vi "Convert X & Y to polar degrees 0 to 360.vi"(8 "error in (no error)":errorcluster, 9 "y":dbl format="%0.2f", 11 "x":dbl format="%0.2f") -> (0 "error out":errorcluster, 2 "degree CCW x axis":dbl, 3 "R":dbl format="%0.2f")   [LabVIEW 2011]
doc: "Does conversion of x and y to polar, with angle in deg and wiht ranbge 0 to 360 CCW from x axis."
uses:
  <vilib>/ptbypt/NI_PtbyPt.lvlib
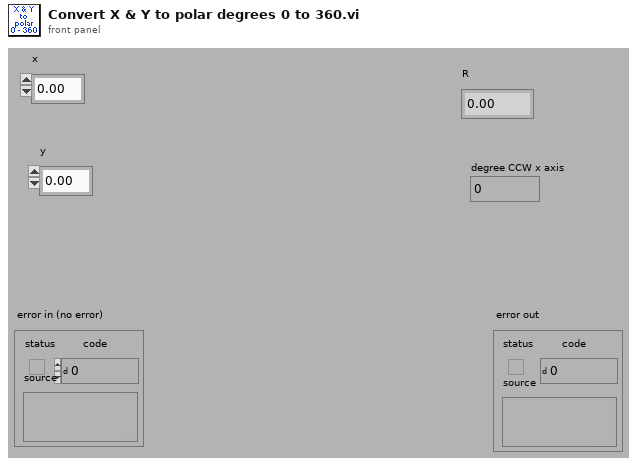
[diagram p1: front panel]
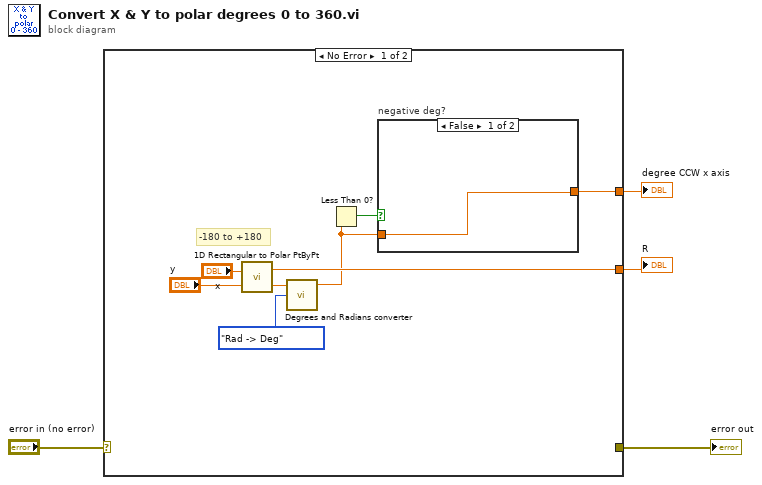
[diagram p0: block diagram]
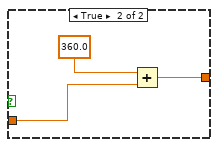
[diagram p2: hidden frame]
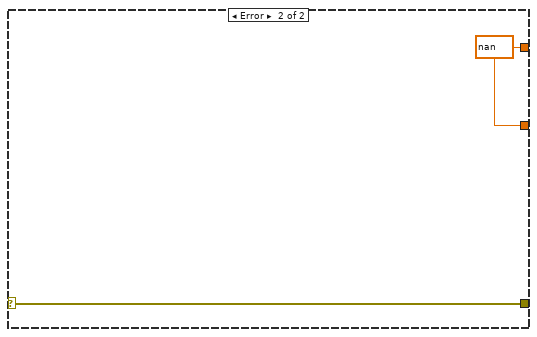
[diagram p3: hidden frame]
diagram:
  n1 = case shown="No Error" "error in (no error)" {
    selector: "error in (no error)" -> [_ w18]
    tunnel: [_ w18] -> w3
    tunnel: [w8 w17] -> w2
    tunnel: [w5 w17] -> w1
    frame No Error {
      # "-180 to +180"
      n2 = call <vilib>:"1D Rectangular to Polar PtByPt.vi"("y"="y", "x"="x") -> ("phase"=w12:dbl, "magnitude"=w8:dbl)
      n3 = call "Degrees and Radians converter.vi"("Units"=enum16{"Deg -> Rad", "Rad -> Deg"}."Rad -> Deg", "Angle IN"=w12) -> ("Angle Out"=w6:dbl)  [unwired: 3 in]
      n4 = Less Than 0?(x=w6) -> (x < 0?=w7:bool)
      n5 = case "negative deg?" shown="False" w7 {
        tunnel: w6 -> [w13 w16]
        tunnel: [w13 w14] -> w5
        frame False {
        }
        frame True {
          n6 = Add(x=360.0 ("y"), y=w16) -> (x+y=w14:dbl)
        }
      }
    }
    frame Error {
      w17 = nan ("Angle Out")
    }
  }
  "error out" <- w3
  "R" <- w2
  "degree CCW x axis" <- w1
